vi "例程26-测量数据的读取.vi"() -> ()   [LabVIEW 2016]
panel:
  out "Signals":dynamicdata(graph) caption="信号"
  out "Comment":string caption="注释"
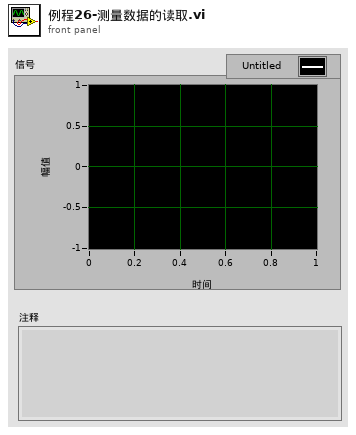
[diagram p1: front panel]
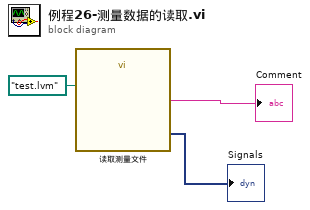
[diagram p0: block diagram]
diagram:
  n1 = call "读取测量文件"("Filename"=path "test.lvm") -> ("Signals"=→"Signals":dynamicdata, "Comment"=→"Comment":string)  [unwired: 5 in, 4 out]
